vi "Write transfer config.vi"(8 "error in (no error)":errorcluster, 10 "transfer config":T1, 11 "Runtime.Transfer in":refnum<class "Runtime.Transfer.lvclass">) -> (0 "error out":errorcluster, 3 "Runtime.Transfer out":refnum<class "Runtime.Transfer.lvclass">)   [LabVIEW 2016, in "Data Sharing Framework.Runtime.lvlib" / "Runtime.Transfer.lvclass"]
uses:
  Runtime.Transfer.lvclass
  Typedefs/Transfer Config.ctl
  Typedefs/Transfer Direction.ctl
  Typedefs/Decimation Factors.ctl
  Runtime.Transfer.lvclass/Runtime.Transfer.ctl
  Data Sharing Framework.Configuration.lvlib
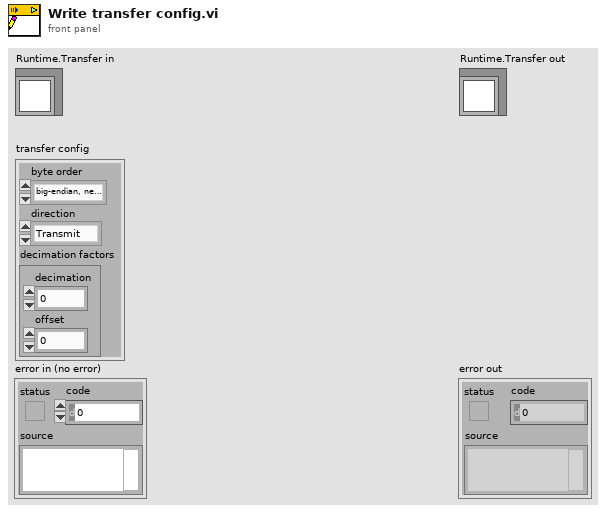
[diagram p1: front panel]
types:
  T1 = typedef "Data Sharing Framework.Configuration.lvlib/Transfer Config.ctl" = cluster{"byte order":enum16{"big-endian, network order", "native, host order", "little-endian"}, "direction":T2, "decimation factors":T3}
  T2 = typedef "Data Sharing Framework.Configuration.lvlib/Transfer Direction.ctl" = enum16{"Transmit", "Receive"}
  T3 = typedef "Data Sharing Framework.Configuration.lvlib/Decimation Factors.ctl" = cluster{"decimation":u16, "offset":u16}
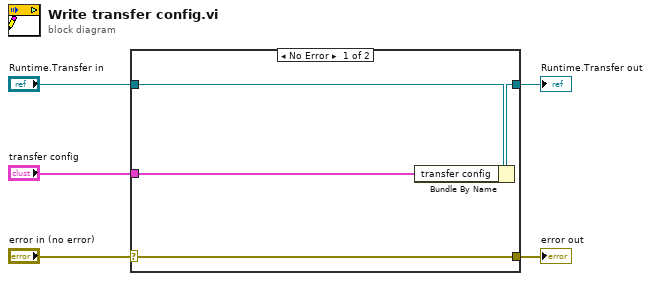
[diagram p0: block diagram]
diagram:
  n1 = case shown="No Error" "error in (no error)" {
    selector: "error in (no error)" -> [w9 w10]
    tunnel: [w9 w10] -> w4
    tunnel: [w7 w11] -> w2
    tunnel: "Runtime.Transfer in" -> [w8 w11]
    tunnel: "transfer config" -> [w6 _]
    frame No Error {
      n2 = Bundle By Name(cluster=w8, "transfer config"=w6) -> (w7:refnum<class "Runtime.Transfer.lvclass">)
    }
    frame Error {
    }
  }
  "error out" <- w4
  "Runtime.Transfer out" <- w2
